vi "Frisbee Counter.vi"(0 "Frisbee States":T1) -> (1 "frisbee counter":i16, 2 "Stack Empty?":bool, 3 "Stack Full?":bool)   [LabVIEW 2012]
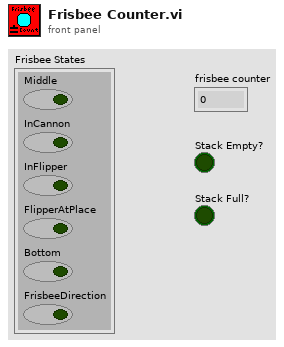
[diagram p1: front panel]
types:
  T1 = cluster{"Middle":bool, "InCannon":bool, "InFlipper":bool, "FlipperAtPlace":bool, "Bottom":bool, "FrisbeeDirection":bool}
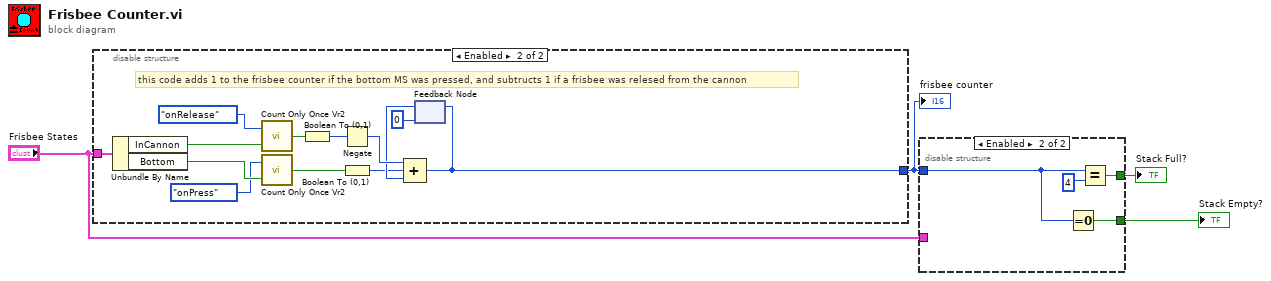
[diagram p0: block diagram]
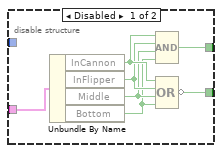
[diagram p2: hidden frame]
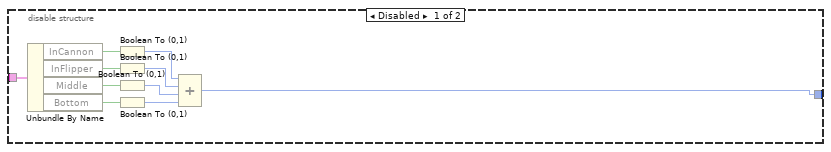
[diagram p3: hidden frame]
diagram:
  n1 = disable-structure shown="Enabled" {
    disable-tunnel: "Frisbee States" -> [w14 w27]
    disable-tunnel: [w5 w15] -> w1
    frame Disabled {
      n2 = Unbundle By Name(w14) -> ("InCannon"=w13:bool, "InFlipper"=w12:bool, "Middle"=w11:bool, "Bottom"=w10:bool)
      n3 = Boolean To (0,1)(Boolean=w13) -> (0, 1=w9:i16)
      n4 = Boolean To (0,1)(Boolean=w12) -> (0, 1=w8:i16)
      n5 = Boolean To (0,1)(Boolean=w11) -> (0, 1=w7:i16)
      n6 = Boolean To (0,1)(Boolean=w10) -> (0, 1=w6:i16)
      n7 = Compound Arithmetic op=ADD(w9, w8, w7, w6) -> (w5:i16)
    }
    frame Enabled {
      # "this code adds 1 to the frisbee counter if the bottom MS was pressed, and subtructs 1 if a frisbee was relesed from the cannon"
      n8 = Unbundle By Name(w27) -> ("InCannon"=w23:bool, "Bottom"=w26:bool)
      n9 = call "Count Only Once Vr2.vi"("InValue"=w23, "Action"=enum16{"onPress", "onRelease", "Both"}."onRelease") -> ("Result"=w21:bool)
      n10 = call "Count Only Once Vr2.vi"("InValue"=w26, "Action"=enum16{"onPress", "onRelease", "Both"}."onPress") -> ("Result"=w25:bool)
      n11 = Boolean To (0,1)(Boolean=w21) -> (0, 1=w20:i16)
      n12 = Negate(x=w20) -> (-x=w19:i16)
      n13 = Boolean To (0,1)(Boolean=w25) -> (0, 1=w17:i16)
      n14 = feedback #1(i16 0) -> (w18:i16)
      n15 = Compound Arithmetic op=ADD(w19, w17, w18) -> (w15:i16)
      n16 = feedback-in #1(w15) -> ()
    }
  }
  "frisbee counter" <- w1
  n17 = disable-structure shown="Enabled" {
    disable-tunnel: "Frisbee States" -> [w30 _]
    disable-tunnel: [w29 w37] -> w3
    disable-tunnel: [w28 w35] -> w2
    disable-tunnel: w1 -> [_ w36]
    frame Disabled {
      n18 = Unbundle By Name(w30) -> ("InCannon"=w34:bool, "InFlipper"=w33:bool, "Middle"=w32:bool, "Bottom"=w31:bool)
      n19 = Compound Arithmetic op=AND(w34, w33, w32, w31) -> (w29:bool)
      n20 = Compound Arithmetic op=OR(w34, w33, w32, w31) -> (invert w28:bool)
    }
    frame Enabled {
      n21 = Equal To 0?(x=w36) -> (x = 0?=w35:bool)
      n22 = Equal?(x=w36, y=i16 4) -> (x = y?=w37:bool)
    }
  }
  "Stack Full?" <- w3
  "Stack Empty?" <- w2
